vi "AcquireData.vi"(8 "error in (no error)":errorcluster, 11 "923x acquisition config":T5={"Acq"=FALSE, "NumberOfModules"=0, "Dynamic FPGA VI Ref"=refnum, "KeyphasorX3"=[], "FixedSizeX32"={"EnabledChannels"=[], "Sensitivity"=[], "InputConfig"=[]}, "SamplingInfo"={"Number of Channels"=4, "Sampling Rate"=4.0, "Channels"=[], "Units"=[], "Offsets"=[]}, "Normal Mode Sample Rate"=0.0, "BlockSize (sec)"=0.0, "Samples To Read (per chan)"=0, "RunningAcquisitionLength"=0.0, "Settling Time"=0.0, "Waveform Groups"=[], "Acquisition Block Number"=0, "Device Name"="", "ValidConfig"=FALSE, "Last Dynamic Module"="", "HighPassFilterState"=[], "Low Frequency Cutoff"=[], "BurstMode"={"Acquisition Time"=0.0, "Sample Rate"=0.0}} {"HighPassFilterState"."Filter State" format="%.2f"; "HighPassFilterState"."IIR Filter Cluster"."Forward Coefficients" format="%.2f"; "HighPassFilterState"."IIR Filter Cluster"."Reverse Coefficients" format="%.2f"; "FixedSizeX32"."InputConfig" items=["AC Coupled", "DC Coupled", "IEPE AC Coupled"]}) -> (0 "error out":errorcluster, 1 "dataflow messages":T1[](array[typedef]), 3 "923x acquisition config out":T5={"Acq"=FALSE, "NumberOfModules"=0, "Dynamic FPGA VI Ref"=refnum, "KeyphasorX3"=[], "FixedSizeX32"={"EnabledChannels"=[], "Sensitivity"=[], "InputConfig"=[]}, "SamplingInfo"={"Number of Channels"=4, "Sampling Rate"=4.0, "Channels"=[], "Units"=[], "Offsets"=[]}, "Normal Mode Sample Rate"=0.0, "BlockSize (sec)"=0.0, "Samples To Read (per chan)"=0, "RunningAcquisitionLength"=0.0, "Settling Time"=0.0, "Waveform Groups"=[], "Acquisition Block Number"=0, "Device Name"="", "ValidConfig"=FALSE, "Last Dynamic Module"="", "HighPassFilterState"=[], "Low Frequency Cutoff"=[], "BurstMode"={"Acquisition Time"=0.0, "Sample Rate"=0.0}} {"HighPassFilterState"."Filter State" format="%.2f"; "HighPassFilterState"."IIR Filter Cluster"."Forward Coefficients" format="%.2f"; "HighPassFilterState"."IIR Filter Cluster"."Reverse Coefficients" format="%.2f"; "FixedSizeX32"."InputConfig" items=["AC Coupled", "DC Coupled", "IEPE AC Coupled"]})   [LabVIEW 2017, in "CmsAcquisition.lvlib"]
uses:
  <vilib>/addons/InsightCM/Devices/Shared/Cms/CmsAcquisition/CmsAcquisition.lvlib
  <vilib>/addons/InsightCM/Devices/Shared/Cms/CmsAcquisition/controls/Configuration.ctl
  <vilib>/addons/InsightCM/Devices/Shared/Cms/CmsAcquisition/controls/TachometerConfig.ctl
  <vilib>/addons/InsightCM/Devices/Shared/Cms/CmsAcquisition/controls/FixedSizeArrays.ctl
  <vilib>/LabVIEW Targets/FPGA/cRIO/shared/nicrio_ModuleControls/nicrio_cRIO-9232_ConfigModeRing.ctl
  <vilib>/addons/InsightCM/Devices/Shared/Cms/cRIOWfmAcq/subVIs/RIO Wfm Cust Ctrls/rwfm_SamplingInfo.ctl
  <vilib>/addons/InsightCM/Devices/Shared/Cms/CmsAcquisition/controls/Group.ctl
  <vilib>/addons/InsightCM/Devices/Shared/Cms/CmsAcquisition/controls/Channel.ctl
  <vilib>/addons/InsightCM/Utilities/Analysis/Vibration/controls/HighPassFilterState.ctl
  <vilib>/addons/InsightCM/Devices/Shared/Cms/CmsAcquisition/controls/BurstMode.ctl
  <vilib>/addons/InsightCM/Devices/Shared/Common/DataFlow/controls/Data.ctl
  <vilib>/addons/InsightCM/Utilities/DataAccessors/controls/wfmSGL_DVR.ctl
  <vilib>/addons/PointValueMap/controls/PointMap.ctl
  <vilib>/addons/InsightCM/Devices/Shared/Common/DataFlow/controls/Type.ctl
  <vilib>/addons/PointValueMap/PointValueMap.lvlib
  <vilib>/addons/InsightCM/Devices/Shared/Common/DataFlow/DataFlow.lvlib
  <vilib>/addons/InsightCM/Devices/Shared/Cms/cRIOWfmAcq/cRIOWfmLib.lvlib
  <vilib>/addons/InsightCM/Utilities/Analysis/Vibration/VibrationAnalysisFunctions.lvlib
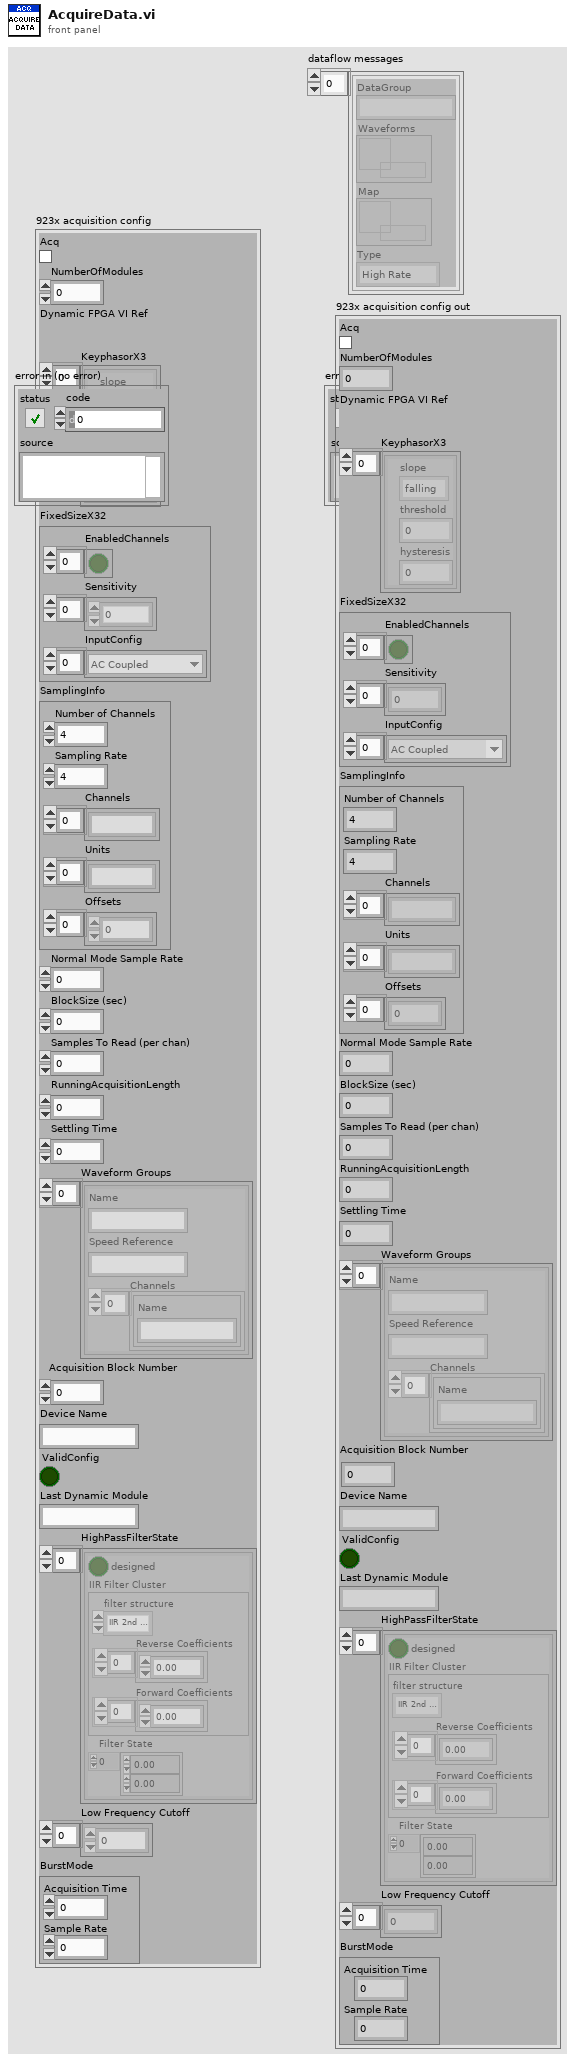
[diagram p1: front panel]
types:
  T1 = typedef "DataFlow.lvlib/Data.ctl" = cluster{"DataGroup":string, "Waveforms":T2, "Map":T3, "Type":T4}
  T2 = typedef "wfmSGL_DVR.ctl" = refnum<data-value>
  T3 = typedef "PointValueMap.lvlib/PointMap.ctl" = refnum<data-value>
  T4 = typedef "DataFlow.lvlib/Type.ctl" = enum16{"High Rate", "Low Rate", "Burst Mode"}
  T5 = typedef "CmsAcquisition.lvlib/Configuration.ctl" = cluster{"Acq":bool, "NumberOfModules":i16, "Dynamic FPGA VI Ref":refnum<k20>, "KeyphasorX3":T6[], "FixedSizeX32":T7, "SamplingInfo":T9, "Normal Mode Sample Rate":dbl, "BlockSize (sec)":dbl, "Samples To Read (per chan)":i32, "RunningAcquisitionLength":dbl, "Settling Time":dbl, "Waveform Groups":T10[], "Acquisition Block Number":i32, "Device Name":string, "ValidConfig":bool, "Last Dynamic Module":string, "HighPassFilterState":T12[], "Low Frequency Cutoff":dbl[], "BurstMode":T13}
  T6 = typedef "CmsAcquisition.lvlib/TachometerConfig.ctl" = cluster{"slope":enum16{"falling", "rising"}, "threshold":dbl, "hysteresis":dbl}
  T7 = typedef "CmsAcquisition.lvlib/FixedSizeArrays.ctl" = cluster{"EnabledChannels":bool[], "Sensitivity":dbl[], "InputConfig":T8[]}
  T8 = typedef "nicrio_cRIO-9232_ConfigModeRing.ctl" = u8
  T9 = typedef "cRIOWfmLib.lvlib/rwfm_SamplingInfo.ctl" = cluster{"Number of Channels":i32, "Sampling Rate":dbl, "Channels":string[], "Units":string[], "Offsets":sgl[]}
  T10 = typedef "CmsAcquisition.lvlib/Group.ctl" = cluster{"Name":string, "Speed Reference":string, "Channels":T11[]}
  T11 = typedef "CmsAcquisition.lvlib/Channel.ctl" = cluster{"Name":string}
  T12 = typedef "VibrationAnalysisFunctions.lvlib/HighPassFilterState.ctl" = cluster{"designed":bool, "IIR Filter Cluster":cluster{"filter structure":enum32{"IIR 2nd Order", "IIR 4th Order"}, "Reverse Coefficients":dbl[], "Forward Coefficients":dbl[]}, "Filter State":dbl[]}
  T13 = typedef "CmsAcquisition.lvlib/BurstMode.ctl" = cluster{"Acquisition Time":dbl, "Sample Rate":dbl}
  T14 = typedef "AnalysisHelper.lvlib/PulsePositions.ctl" = cluster{"Name":string, "Pulse Position Data":dbl[], "Pulses Per Rev":i32}
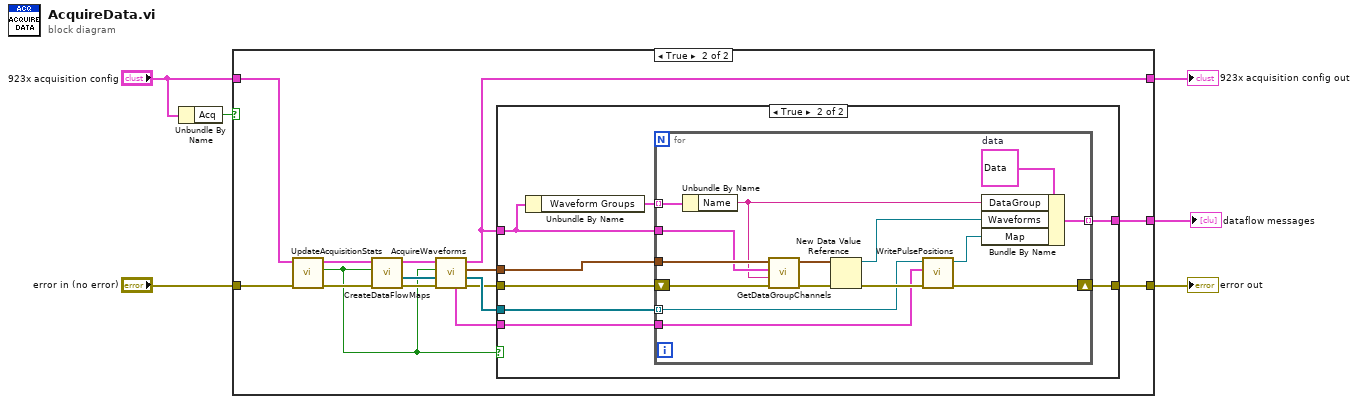
[diagram p0: block diagram]
diagram:
  n1 = Unbundle By Name("923x acquisition config") -> ("Acq"=w1:bool)
  n2 = case shown="True" w1 {
    tunnel: "923x acquisition config" -> [w8 w23]
    tunnel: [w8 w11] -> w6
    tunnel: [w7 w17] -> w5
    tunnel: [_ w16] -> w4
    tunnel: "error in (no error)" -> [w7 w15]
    frame False {
    }
    frame True {
      n3 = call <vilib>:"UpdateAcquisitionStats.vi"("error in (no error)"=w15, "configuration"=w23) -> ("error out"=w22:errorcluster, "settling time requirement met?"=w14:bool, "configuration"=w13:T5)  [unwired: 7 in]
      n4 = call <vilib>:"CreateDataFlowMaps.vi"("error in (no error)"=w22, "settling time met"=w14, "923x Acquisition Config"=w13) -> ("error out"=w19:errorcluster, "maps"=w21:T3[], "923x Acquisition Config out"=w12:T5)  [unwired: 6 in]
      n5 = call <vilib>:"AcquireWaveforms.vi"("error in (no error)"=w19, "Data Flow Maps"=w21, "settling time met"=w14, "923x Acquisition Config"=w12) -> ("error out"=w18:errorcluster, "Data Flow Maps out"=w20:T3[], "Waveforms"=w10:waveform(sgl)[], "923x Acquisition Config out"=w11:T5, "Pulse Positions Array"=w9:T14[])  [unwired: 3 in]
      n6 = case shown="True" w14 {
        tunnel: w20 -> [_ w32]
        tunnel: w18 -> [w24 w31]
        tunnel: [w24 w30] -> w17
        tunnel: [_ w29] -> w16
        tunnel: w9 -> [_ w28]
        tunnel: w10 -> [_ w27]
        tunnel: w11 -> [_ w26]
        frame False {
        }
        frame True {
          n7 = Unbundle By Name(w26) -> ("Waveform Groups"=w25:T10[])
          n8 = for {
            tunnel: w25 -> [w35] mode=indexing
            tunnel: w27 -> [w36]
            tunnel: w28 -> [w43]
            tunnel: w32 -> [w40] mode=indexing
            tunnel: [w47] -> w29 mode=indexing
            shift-right: [w41] -> w30
            shift-left: w31 -> [w38]
            tunnel: w26 -> [w34]
            w46 = T1 {"DataGroup"="", "Waveforms"=refnum, "Map"=refnum, "Type"=enum."High Rate"}  # data
            n9 = Unbundle By Name(w35) -> ("Name"=w33:string)
            n10 = call <vilib>:"GetDataGroupChannels.vi"("error in (no error)"=w38, "group"=w33, "923x acquisition config"=w34, "all waveforms"=w36) -> ("error out"=w39:errorcluster, "this groups channels"=w37:waveform(sgl)[])  [unwired: 6 in]
            n11 = New Data Value Reference(data value=w37, error in=w39) -> (data value reference=w45:refnum<data-value>, error out=w44:errorcluster)
            n12 = call <vilib>:"WritePulsePositions.vi"("error in (no error)"=w44, "pulse positions array"=w43, "map in"=w40) -> ("error out"=w41:errorcluster, "map out"=w42:T3)  [unwired: 7 in]
            n13 = Bundle By Name(cluster=w46, "DataGroup"=w33, "Waveforms"=w45, "Map"=w42) -> (w47:T1)
          }
        }
      }
    }
  }
  "error out" <- w5
  "923x acquisition config out" <- w6
  "dataflow messages" <- w4
